vi "Nest Msg Send.vi"(8 "Alias":string, 9 "Msg EnQ":refnum<class "Msg EnQ.lvclass">, 10 "Msg":refnum<class "Msg.lvclass">, 11 "Self Actor in":refnum<class "Self Actor.lvclass">) -> (0 "error out":errorcluster)   [LabVIEW 2021, in "AAM.lvlib" / "Self Actor.lvclass"]
uses:
  Self Actor.lvclass
  Msg Q/Msg Q.lvclass
  Msg EnQ/Msg EnQ.lvclass
  Msg/Msg.lvclass
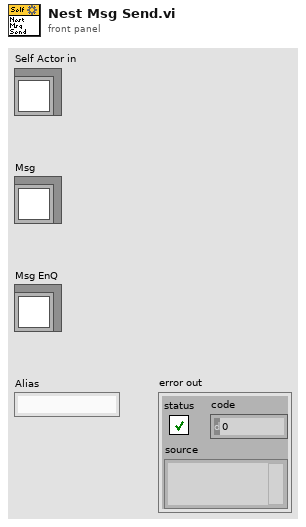
[diagram p1: front panel]
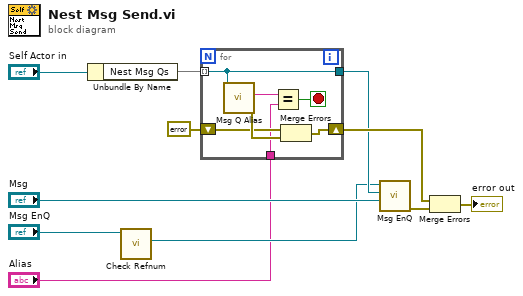
[diagram p0: block diagram]
diagram:
  n1 = Unbundle By Name("Self Actor in") -> ("Nest Msg Qs"=w10:set{refnum<class "Msg Q.lvclass">})
  n2 = call "Check Refnum.vi"("Msg EnQ in"="Msg EnQ") -> ("Msg EnQ out"=w2:refnum<class "Msg EnQ.lvclass">)  [unwired: 10 in]
  n3 = for {
    tunnel: w10 -> [w17] mode=indexing
    tunnel: "Alias" -> [w12]
    tunnel: [w17] -> w4
    shift-right: [w15] -> w5
    shift-left: errorcluster {"status"=FALSE, "code"=0, "source"=""} ("error out") -> [w14]
    stop <- w18 stop-if-true
    n4 = call "Msg Q Alias.vi"("Msg Q in"=w17) -> ("error out"=w16:errorcluster, "Msg Q Alias"=w13:string)  [unwired: 9 in]
    n5 = Equal?(x=w13, y=w12) -> (x = y?=w18:bool)
    n6 = Merge Errors(w14, w16) -> (w15:errorcluster)
  }
  n7 = call-dynamic "Msg EnQ.vi"("Msg"="Msg", "Msg Q"=w4, "Msg EnQ in"=w2) -> ("error out"=w6:errorcluster)  [unwired: 8 in]
  n8 = Merge Errors(w5, w6) -> (→"error out":errorcluster)
